vi "ASI Cavity Scan V1.vi"() -> ()   [LabVIEW 2014]
uses:
  ROI Action.ctl
  Controls/StageStates.ctl
  <vilib>/Analysis/baseanly.llb/Mean (DBL).vi
  <vilib>/Analysis/NI_AALBase.lvlib
panel:
  out "Current Position (µm)":dbl=1.0
  in  "Clear ROIs":bool
  in  "Abort":bool
  out "Scan Plot":cluster{dbl[], dbl[]}[](graph)
  in  "Scan Speed (µm/sec)":dbl=1.0
  in  "Scan Range (µm)":dbl
  in  "ROI Size (px)":u8(slide)=4 min=2 step=1 scale=2.0..50.0
  in  "Add ROIs":bool
  in  "Scan":bool
  in  "Exit":bool
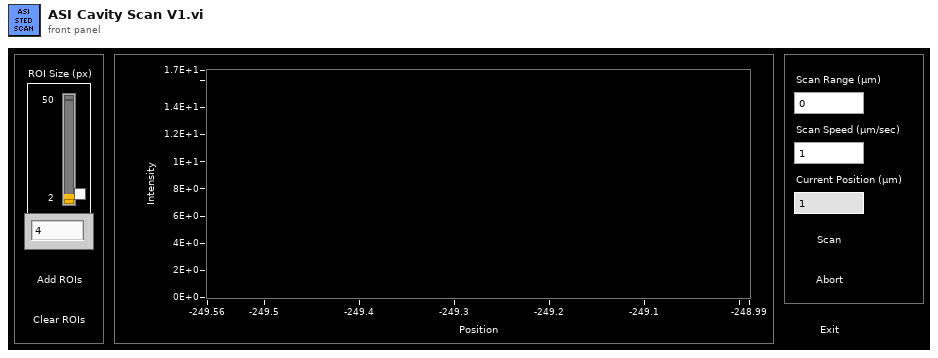
[diagram p1: front panel]
types:
  T1 = typedef "StageStates.ctl" = enum16{"POSITION", "MVR", "MOVE", "HALT", "ONTARGET", "ERROR", "EXIT", "HOME", "ZEROPOS", "NANOPOS", "QUIT", "ANALOG"}
  T2 = typedef "ROI Action.ctl" = enum16{"Reset", "Add New ROI", "Resize ROIs", "Get ROI Indices"}
  T3 = typedef "Image Acquisition Parameters.ctl" = cluster{"Scan Type":enum16{"Sample Scanning", "Beam Scanning"}, "Scan Mode":enum16{"XY", "XZ", "YZ", "XYZ"}, "Fast Axis Frequency (Hz)":dbl, "Image Format":u16, "Line Accumulations":u16, "Frames Per Capture":u16, "Frames Accumulations":u16, "Image Dimension (um)":dbl[], "Number of Z Steps":u8, "Z Steps Size (um)":dbl, "Pixel Size (nm)":dbl[]}
  T4 = typedef "IMAQ Image.ctl" = refnum<image>
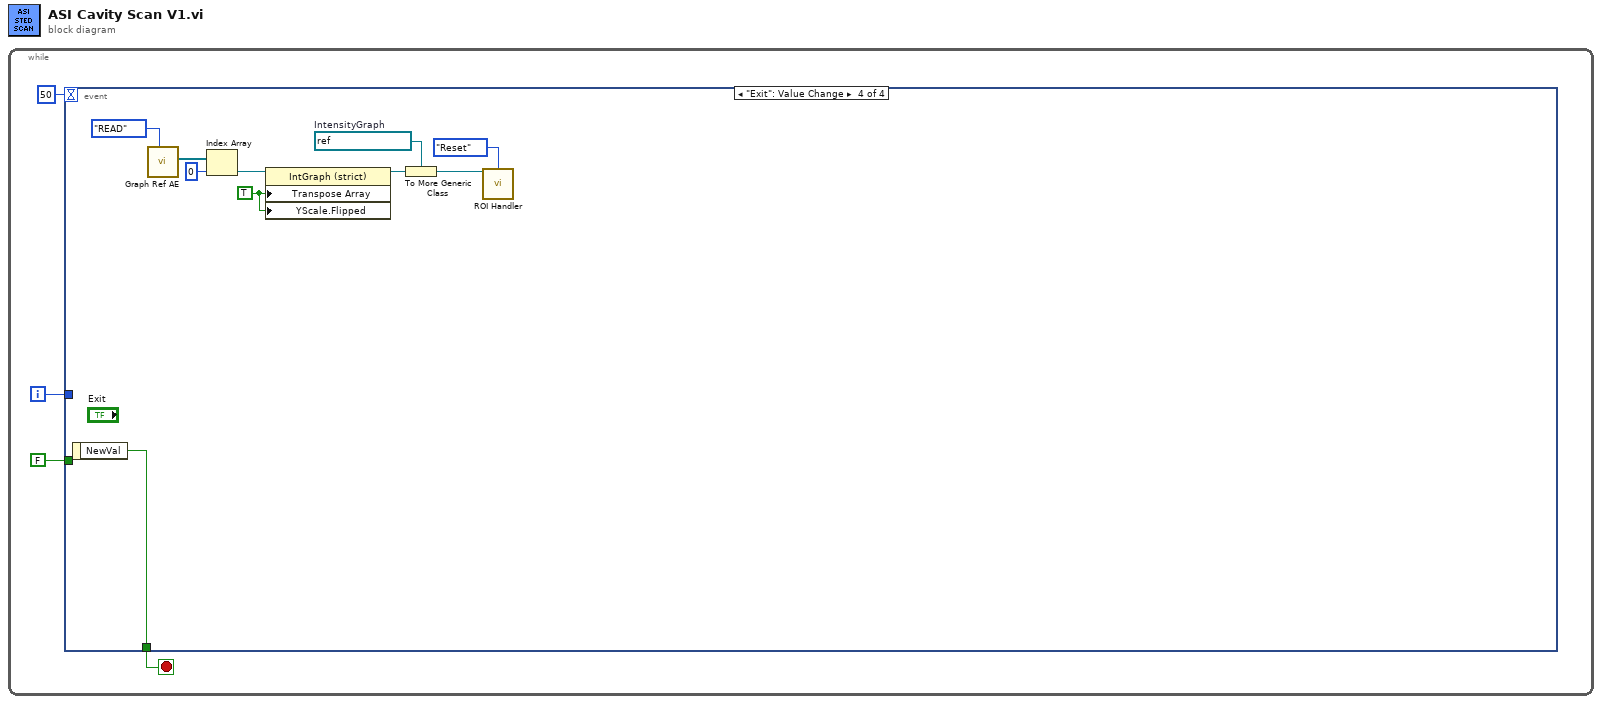
[diagram p0: block diagram]
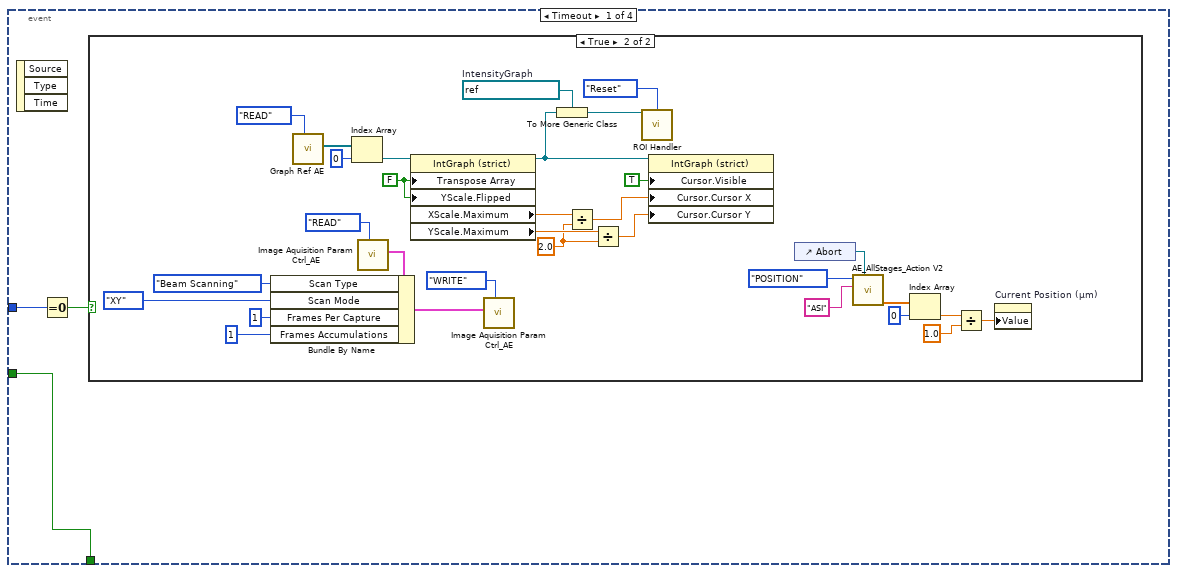
[diagram p2: hidden frame]
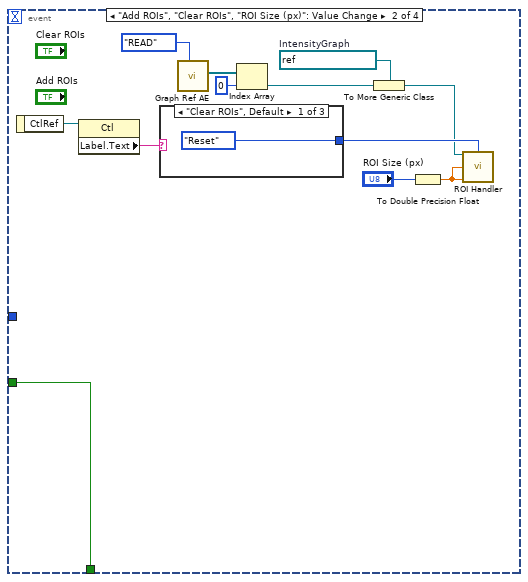
[diagram p4: hidden frame]
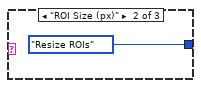
[diagram p5: hidden frame]
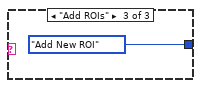
[diagram p6: hidden frame]
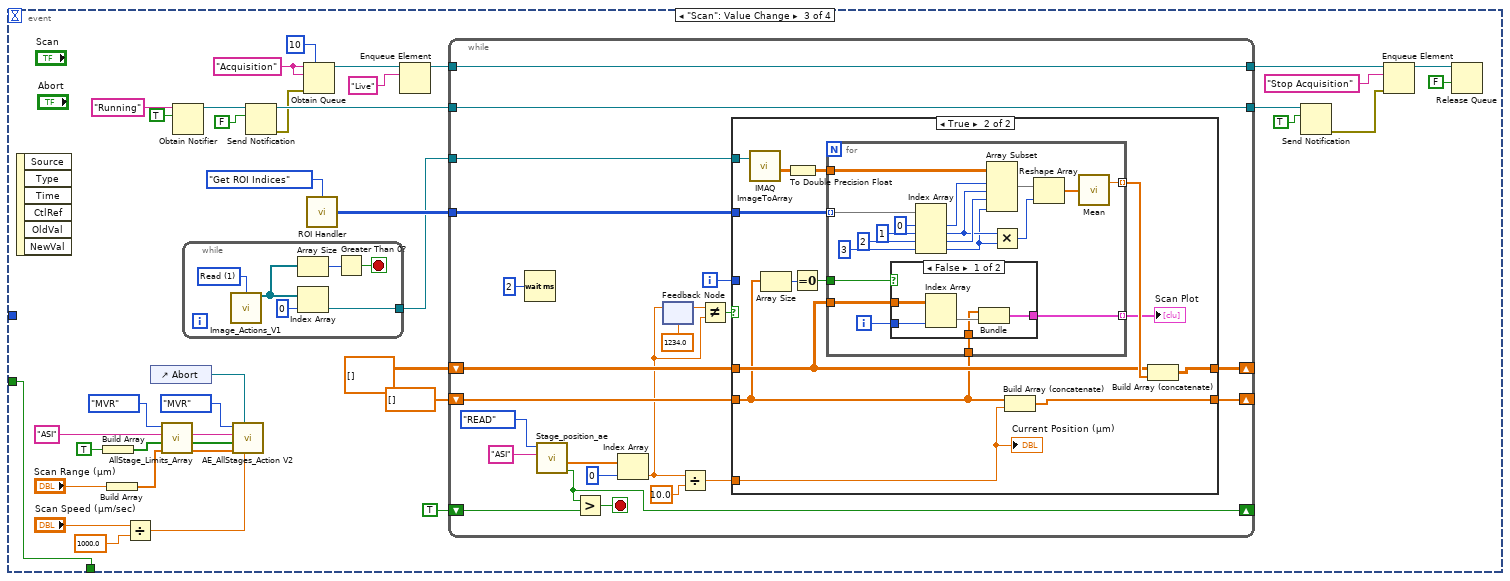
[diagram p7: hidden frame]
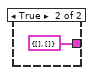
[diagram p9: hidden frame]
diagram:
  n1 = while {
    i -> [w1]
    stop <- w2 stop-if-true
    n2 = event shown="[3] \"Exit\": Value Change" {
      selector: _ -> [_ _ _ _]
      dyn-events: _ -> [_ _ _ _]
      timeout: 50 -> [_ _ _ _]
      tunnel: [w5 w50 w54 w171] -> w2
      tunnel: FALSE -> [w5 w50 w54 _]
      tunnel: w1 -> [w6 _ _ _]
      event Timeout {
        n3 = event-data() -> ()  [unwired: 1 in, 3 out]
        n4 = Equal To 0?(x=w6) -> (x = 0?=w7:bool)
        n5 = case shown="True" w7 {
          frame False {
          }
          frame True {
            w20 = 2.0 ("y")
            w24 = FALSE ("Transpose Array")
            w30 = refnum<vi> refnum  # IntensityGraph
            n6 = call "Graph Ref AE.vi"("Action"=enum16{"READ", "WRITE"}."READ") -> ("Graph Ref Out"=w27:refnum<vi>[])  [unwired: 10 in]
            n7 = Index Array(array=w27, index=0) -> (element=w25:refnum<vi>)
            n8 = call "Image Aquisition Param Ctrl_AE.vi"("Action"=enum16{"READ", "WRITE"}."READ") -> ("Image Acquisition Parameters Out"=w37:T3)  [unwired: 10 in]
            n9 = Bundle By Name(cluster=w37, "Scan Type"=enum16{"Sample Scanning", "Beam Scanning"}."Beam Scanning", "Scan Mode"=enum16{"XY", "XZ", "YZ", "XYZ"}."XY", "Frames Per Capture"=u16 1, "Frames Accumulations"=u16 1) -> (w35:T3)
            n10 = property class="IntGraph (strict)"(reference=w25, "Transpose Array"=w24, "YScale.Flipped"=w24) -> (reference out=w18:refnum<vi>, "XScale.Maximum"=w22:dbl, "YScale.Maximum"=w21:dbl)  [unwired: 1 in, 1 out]
            n11 = call "Image Aquisition Param Ctrl_AE.vi"("Action"=enum16{"READ", "WRITE"}."WRITE", "Image Acquisition Parameters In"=w35) -> ()  [unwired: 9 in, 1 out]
            n12 = To More Generic Class(target class=w30, reference=w18) -> (generic class reference=w29:refnum<vi>)
            n13 = Divide(x=w22, y=w20) -> (x/y=w16:dbl)
            n14 = Divide(x=w21, y=w20) -> (x/y=w17:dbl)
            n15 = call "ROI Handler.vi"("IntGraph REF"=w29, "ROI Action"=ROI_Action."Reset") -> ()  [unwired: 12 in, 2 out]
            n16 = property class="IntGraph (strict)"(reference=w18, "Cursor.Visible"=TRUE, "Cursor.Cursor X"=w16, "Cursor.Cursor Y"=w17) -> ()  [unwired: 1 in, 2 out]
            n17 = control-ref of="Abort"() -> (w11:refnum<vi>)
            n18 = call "AE_AllStages_Action V2.vi"("Abort"=w11, "Stage ID"="ASI", "Action"=StageStates."POSITION") -> ("Position Out"=w14:dbl[])  [unwired: 6 in, 2 out]
            n19 = Index Array(array=w14, index=0) -> (element=w10:dbl)
            n20 = Divide(x=w10, y=1.0) -> (x/y=w9:dbl)
            n21 = property on="Current Position (µm)" class="DigNum (strict)"("Value"=w9) -> ()  [unwired: 2 in, 2 out]
          }
        }
      }
      event "Add ROIs", "Clear ROIs", "ROI Size (px)": Value Change {
        w44 = refnum<vi> refnum  # IntensityGraph
        n22 = event-data() -> ("CtlRef"=w49:refnum<vi>)  [unwired: 1 in]
        n23 = property class="Ctl"(reference=w49) -> ("Label.Text"=w48:string)  [unwired: 1 in, 2 out]
        n24 = case shown="\"Clear ROIs\", Default" w48 {
          tunnel: [ROI_Action."Reset" ("ROI Action") ROI_Action."Resize ROIs" ("ROI Action") ROI_Action."Add New ROI" ("ROI Action")] -> w47
          frame "Clear ROIs", Default {
          }
          frame "ROI Size (px)" {
          }
          frame "Add ROIs" {
          }
        }
        n25 = call "Graph Ref AE.vi"("Action"=enum16{"READ", "WRITE"}."READ") -> ("Graph Ref Out"=w41:refnum<vi>[])  [unwired: 10 in]
        n26 = Index Array(array=w41, index=0) -> (element=w43:refnum<vi>)
        n27 = To More Generic Class(target class=w44, reference=w43) -> (generic class reference=w39:refnum<vi>)
        n28 = To Double Precision Float(number="ROI Size (px)") -> (double precision float=w45:dbl)
        n29 = call "ROI Handler.vi"("IntGraph REF"=w39, "ROI Action"=w47, "X Width (PX)"=w45, "Y Width (PX)"=w45) -> ()  [unwired: 10 in, 2 out]
      }
      event "Scan": Value Change {
        w63 = "Acquisition" ("name (unnamed)")
        n30 = event-data() -> ()  [unwired: 1 in, 6 out]
        n31 = Build Array(TRUE) -> (w88:bool[])
        n32 = Build Array("Scan Range (µm)") -> (w86:dbl[])
        n33 = Divide(x="Scan Speed (µm/sec)", y=1000.0) -> (x/y=w79:dbl)
        n34 = control-ref of="Abort"() -> (w82:refnum<vi>)
        n35 = call "AllStage_Limits_Array.vi"("Step(um)/Position(units)"=w86, "Axis"=w88, "Stage ID"="ASI", "MOVE/MVR"=enum16{"MOVE", "MVR"}."MVR") -> ("Positions"=w91:dbl[], "Boolean Array"=w90:bool[], "Stage ID"=w89:string)  [unwired: 5 in]
        n36 = Obtain Notifier(name (unnamed)="Running", notification data type=TRUE) -> (notifier out=w68:refnum<notifier>)  [unwired: 2 in, 2 out]
        n37 = while {
          tunnel: [w93] -> w55
          stop <- w94 stop-if-true
          w97 = u16 1 items=["Write", "Read"] ("Mode")
          n38 = call "Image_Actions_V1.vi"("Mode"=w97) -> ("Image REFs OUT"=w96:T4[])  [unwired: 13 in, 1 out]
          n39 = Array Size(array=w96) -> (size(s)=w95:i32)
          n40 = Index Array(array=w96, index=0) -> (element=w93:T4)
          n41 = Greater Than 0?(x=w95) -> (x > 0?=w94:bool)
        }
        n42 = call "AE_AllStages_Action V2.vi"("Velocity"=w79, "Abort"=w82, "Positions"=w91, "Axis"=w90, "Stage ID"=w89, "Action"=StageStates."MVR") -> ()  [unwired: 3 in, 3 out]
        n43 = Send Notification(notification=FALSE, notifier=w68) -> (notifier out=w72:refnum<notifier>, error out=w69:errorcluster)  [unwired: 1 in]
        n44 = Obtain Queue(max queue size (-1, unlimited)=10, name (unnamed)=w63, element data type=w63, error in (no error)=w69) -> (queue out=w65:refnum<queue>)  [unwired: 1 in, 2 out]
        n45 = call "ROI Handler.vi"("ROI Action"=ROI_Action."Get ROI Indices") -> ("ROI Indices OUT"=w77:i32[][])  [unwired: 13 in, 1 out]
        n46 = Enqueue Element(queue=w65, element="Live") -> (queue out=w71:refnum<queue>)  [unwired: 2 in, 2 out]
        n47 = while {
          shift-right: [w104] -> _
          shift-left: TRUE ("Status Out") -> [w116]
          tunnel: w71 -> [w113]
          tunnel: w72 -> [w112]
          tunnel: [w113] -> w73
          tunnel: [w112] -> w74
          shift-right: [w106] -> _
          shift-left: dbl[] [] -> [w105]
          tunnel: w55 -> [w111]
          tunnel: w77 -> [w110]
          shift-right: [w109] -> _
          shift-left: dbl[][] [] -> [w107]
          i -> [w108]
          stop <- w115 stop-if-true
          n48 = Wait (ms)(milliseconds to wait=u32 2) -> ()  [unwired: 1 out]
          n49 = call "Stage_position_ae.vi"("StageID"="ASI", "Enum"=enum16{"WRITE", "READ"}."READ") -> ("Status Out"=w104:bool, "Position Out"=w120:dbl[])  [unwired: 8 in]
          n50 = Greater?(x=w104, y=w116) -> (0:w115:bool)
          n51 = Index Array(array=w120, index=0) -> (element=w99:dbl)
          n52 = feedback-in #1(w99) -> ()
          n53 = feedback #1(1234.0 ("Numeric")) -> (w100:dbl)
          n54 = Divide(x=w99, y=10.0) -> (x/y=w103:dbl)
          n55 = Not Equal?(x=w100, y=w99) -> (x != y?=w101:bool)
          n56 = case shown="True" w101 {
            tunnel: w111 -> [_ w134]
            tunnel: w110 -> [_ w133]
            tunnel: [w123 w131] -> w109
            tunnel: w108 -> [_ _]
            tunnel: w107 -> [w123 w129]
            tunnel: [w122 w128] -> w106
            tunnel: w105 -> [w122 w124]
            tunnel: w103 -> [_ w126]
            frame False {
            }
            frame True {
              n57 = call "IMAQ ImageToArray"("Image"=w134) -> ("Image Pixels (Float)"=w136:sgl[][])  [unwired: 3 in, 4 out]
              n58 = Array Size(array=w124) -> (size(s)=w125:i32)
              n59 = To Double Precision Float(number=w136) -> (double precision float=w135:dbl[][])
              n60 = Equal To 0?(x=w125) -> (x = 0?=w130:bool)
              n61 = for {
                tunnel: w133 -> [w155] mode=indexing
                tunnel: w135 -> [w150]
                tunnel: [w137] -> w132 mode=indexing
                tunnel: w130 -> [w142]
                tunnel: w129 -> [w141]
                tunnel: w124 -> [w139]
                tunnel: [w138] -> w127 mode=indexing
                i -> [w140]
                n62 = case shown="False" w142 {
                  tunnel: w141 -> [w159 _]
                  tunnel: w140 -> [w158 _]
                  tunnel: w139 -> [w157 _]
                  tunnel: [w156 cluster{dbl[], dbl[]} {[], []}] -> w138
                  frame False {
                    n63 = Index Array(array=w159, index (col)=w158) -> (element=w160:dbl[])  [unwired: 1 in]
                    n64 = Bundle(w157, w160) -> (w156:cluster{dbl[], dbl[]})  [unwired: 1 in]
                  }
                  frame True {
                  }
                }
                n65 = Index Array(array=w155, index #1=0 ("index"), index #2=1 ("index"), index #3=2 ("index"), index #4=3 ("index")) -> (element #1=w148:i32, element #2=w146:i32, element #3=w149:i32, element #4=w145:i32)
                n66 = Array Subset(array=w150, index (row)=w148, length (row)=w146, index (col)=w149, length (col)=w145) -> (w147:dbl[][])
                n67 = Multiply(x=w146, y=w145) -> (x*y=w144:i32)
                n68 = Reshape Array(w147, w144) -> (w143:dbl[])
                n69 = call-poly <vilib>:"Mean.vi"("X"=w143) -> ("mean"=w137:dbl)  [unwired: 1 out]
              }
              "Scan Plot" <- w127
              n70 = Build Array (concatenate)(w124, w126) -> (w128:dbl[])
              n71 = Build Array (concatenate)(w129, w132) -> (w131:dbl[][])
              "Current Position (µm)" <- w126
            }
          }
        }
        n72 = Send Notification(notification=TRUE, notifier=w74) -> (error out=w75:errorcluster)  [unwired: 1 in, 1 out]
        n73 = Enqueue Element(queue=w73, element="Stop Acquisition", error in (no error)=w75) -> (queue out=w59:refnum<queue>)  [unwired: 1 in, 2 out]
        n74 = Release Queue(queue=w59, force destroy? (F)=FALSE) -> ()  [unwired: 1 in, 3 out]
      }
      event "Exit": Value Change {
        w164 = refnum<vi> refnum  # IntensityGraph
        w166 = TRUE ("Transpose Array")
        n75 = event-data() -> ("NewVal"=w171:bool)  [unwired: 1 in]
        n76 = call "Graph Ref AE.vi"("Action"=enum16{"READ", "WRITE"}."READ") -> ("Graph Ref Out"=w169:refnum<vi>[])  [unwired: 10 in]
        n77 = Index Array(array=w169, index=0) -> (element=w167:refnum<vi>)
        n78 = property class="IntGraph (strict)"(reference=w167, "Transpose Array"=w166, "YScale.Flipped"=w166) -> (reference out=w163:refnum<vi>)  [unwired: 1 in, 1 out]
        n79 = To More Generic Class(target class=w164, reference=w163) -> (generic class reference=w162:refnum<vi>)
        n80 = call "ROI Handler.vi"("IntGraph REF"=w162, "ROI Action"=ROI_Action."Reset") -> ()  [unwired: 12 in, 2 out]
      }
    }
  }
